vi "SB_fillState.vi"(5 "Water_density [kg/m^3]":dbl=1000.0, 6 "SB_parameters":T1={"x0 [m]"=0.0, "U_full [V]"=3.67, "U_empty [V]"=0.695}, 7 "error in (no error)":errorcluster) -> (0 "x [m]":dbl, 1 "x_norm [-]":dbl, 2 "Percentage_fillState [%]":dbl(slide) scale=0.0..100.0, 3 "error out":errorcluster, 4 "M_y [Nm]":dbl)   [LabVIEW 2013]
uses:
  My Computer/Controls/Advanced Swimbladder Indicators.ctl
  <vilib>/myRIO/Instrument Drivers/Onboard IO/AI/vis/Smart Open.vi
  <vilib>/myRIO/Instrument Drivers/Onboard IO/AI/vis/Read.vi
  <vilib>/myRIO/Instrument Drivers/Onboard IO/AI/vis/Open.vi
  <vilib>/myRIO/Common/Instrument Driver Framework/myRIO v1.0/AI/vis/myRIO v1.1 Open AI.vi
  <vilib>/myRIO/Common/Instrument Driver Framework/Utilities/vis/Validate Channels.vi
  <vilib>/myRIO/Common/Instrument Driver Framework/myRIO v1.0/AI/vis/myRIO v1.0 Reserve AI.vi
  <vilib>/myRIO/Common/Instrument Driver Framework/myRIO v1.0/AI/vis/myRIO v1.0 Build MUX Configuration AI.vi
  <vilib>/myRIO/Common/Instrument Driver Framework/myRIO v1.0/Resource Manager/vis/myRIO v1.0 Reserve Channel List.vi
  <vilib>/myRIO/Common/Instrument Driver Framework/myRIO v1.0/Resource Manager/vis/myRIO v1.0 Reserve Channel.vi
  <vilib>/myRIO/Common/Instrument Driver Framework/myRIO v1.0/Resource Manager/vis/myRIO v1.0 Unreserve Channel.vi
  <vilib>/myRIO/Common/Instrument Driver Framework/myRIO v1.0/Resource Manager/vis/myRIO v1.0 Build Mutex Name.vi
  <vilib>/myRIO/Common/Instrument Driver Framework/myRIO v1.0/myRIO v1.1 Open.vi
  <vilib>/myRIO/Common/Instrument Driver Framework/myRIO v1.0/AI/vis/myRIO v1.0 Get Scaling Constants AI.vi
  <vilib>/Utility/VariantDataType/GetNumericInfo.vi
  <vilib>/Utility/error.llb/Error Cluster From Error Code.vi
  <vilib>/myRIO/Common/Instrument Driver Framework/Utilities/vis/IO Manager.vi
  <vilib>/myRIO/Common/Instrument Driver Framework/Utilities/vis/Configuration Manager.vi
  <vilib>/myRIO/Common/Instrument Driver Framework/myRIO v1.0/myRIO v1.0 Close.vi
  <vilib>/myRIO/Common/Instrument Driver Framework/myRIO v1.0/AI/vis/myRIO v1.0 Read AI.vi
panel:
  out "SB_Voltage":dbl
  # "Current position"
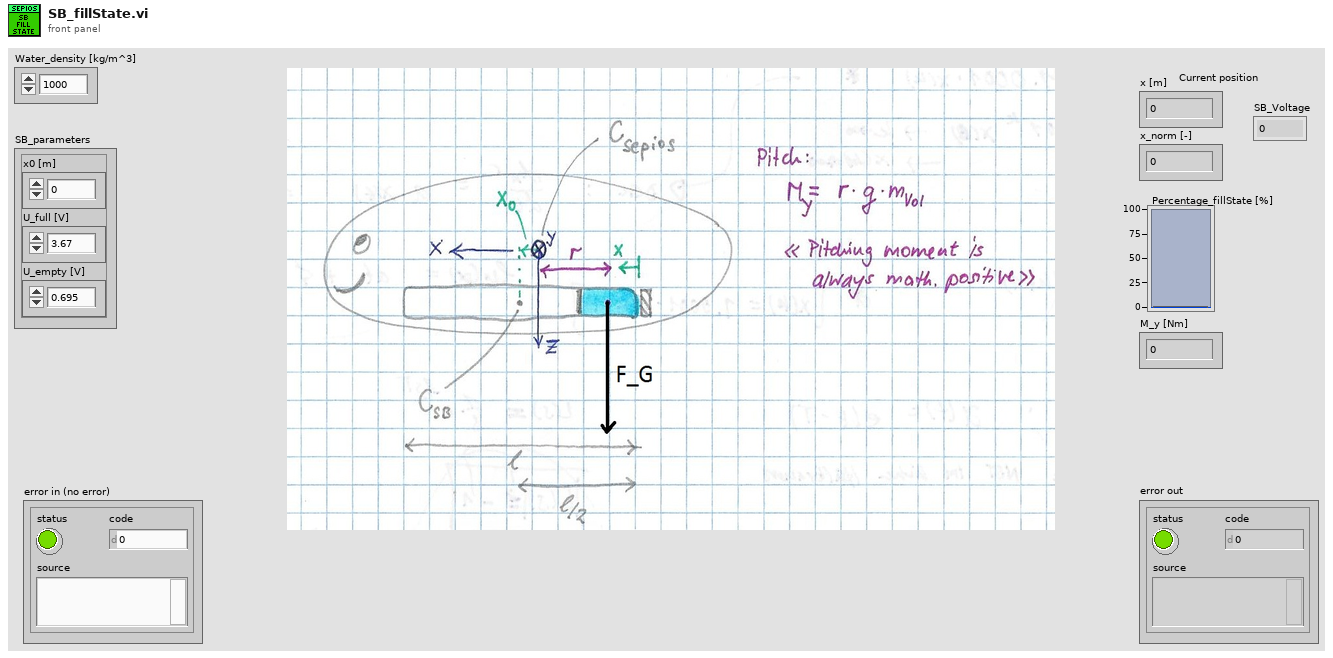
[diagram p1: front panel]
types:
  T1 = cluster{"x0 [m]":dbl, "U_full [V]":dbl, "U_empty [V]":dbl}
  T2 = typedef "Advanced Swimbladder Indicators.ctl" = cluster{"P_ref [Pa]":dbl, "X_Actual [m]":dbl, "Motor Current[A]":dbl}
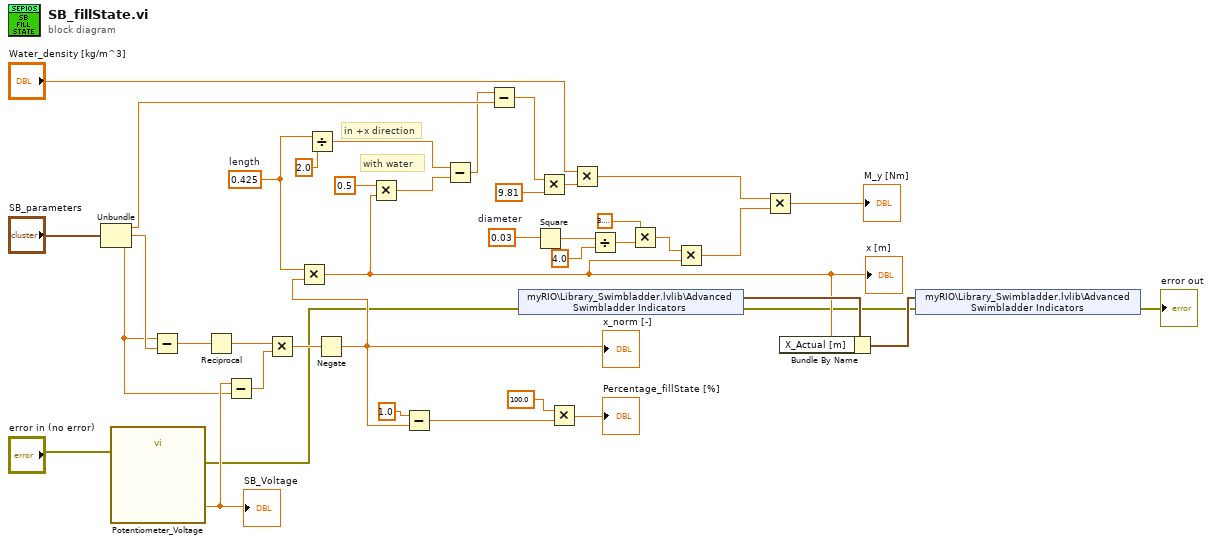
[diagram p0: block diagram]
diagram:
  w23 = 0.03  # diameter
  w30 = 0.425  # length
  # "with water"
  # "in +x direction"
  n1 = Unbundle("SB_parameters") -> ("x0 [m]"=w39:dbl, "U_full [V]"=w12:dbl, "U_empty [V]"=w11:dbl)
  n2 = call "Potentiometer_Voltage"("error in (no error)"="error in (no error)") -> ("SB_POS (A/AI2 (Pin 7))"=w13:dbl, "error out"=w3:errorcluster)  [unwired: 25 in]
  "SB_Voltage" <- w13
  n3 = Subtract(x=w11, y=w12) -> (x-y=w15:dbl)
  n4 = Reciprocal(x=w15) -> (1/x=w17:dbl)
  n5 = Subtract(x=w13, y=w11) -> (x-y=w16:dbl)
  n6 = Multiply(x=w17, y=w16) -> (x*y=w35:dbl)
  n7 = Divide(x=w30, y=2.0) -> (x/y=w32:dbl)
  n8 = Negate(x=w35) -> (-x=w9:dbl)
  "x_norm [-]" <- w9
  n9 = Multiply(x=w30, y=w9) -> (x*y=w4:dbl)
  "x [m]" <- w4
  n10 = Multiply(x=0.5, y=w4) -> (x*y=w20:dbl)
  n11 = Subtract(x=1.0, y=w9) -> (x-y=w10:dbl)
  n12 = Subtract(x=w32, y=w20) -> (x-y=w33:dbl)
  n13 = Subtract(x=w33, y=w39) -> (x-y=w34:dbl)
  n14 = shared-variable "myRIO\\Library_Swimbladder.lvlib\\Advanced Swimbladder Indicators"(error in=w3) -> (w5:T2, error out=w2:errorcluster)
  n15 = Square(x=w23) -> (x^2=w24:dbl)
  n16 = Multiply(x=w34, y=9.81) -> (x*y=w22:dbl)
  n17 = Multiply(x=100.0, y=w10) -> (x*y=→"Percentage_fillState [%]":dbl)
  n18 = Multiply(x="Water_density [kg/m^3]", y=w22) -> (x*y=w27:dbl)
  n19 = Divide(x=w24, y=4.0) -> (x/y=w28:dbl)
  n20 = Multiply(x=3.141592653589793, y=w28) -> (x*y=w7:dbl)
  n21 = Multiply(x=w7, y=w4) -> (x*y=w26:dbl)
  n22 = Multiply(x=w27, y=w26) -> (x*y=→"M_y [Nm]":dbl)
  n23 = Bundle By Name(cluster=w5, "X_Actual [m]"=w4) -> (w6:T2)
  n24 = shared-variable "myRIO\\Library_Swimbladder.lvlib\\Advanced Swimbladder Indicators"(w6, error in=w2) -> (error out=→"error out":errorcluster)
